vi "Get Reference for Demodulation.vi"(0 "AI Block Size":i32=5000, 1 "# channels":i32, 2 "Calculate REF?":bool, 5 "AI Rate":dbl=10000.0 format="%.2f", 7 "OSC Configuration":T3(array[cluster])=[[{"Signal Type"=enum."Sine Wave", "DC"=0.0, "Amplitude"=0.01, "frequency"=2.0, "Phase"=0.0}, {"Signal Type"=enum."Sine Wave", "DC"=0.0, "Amplitude"=0.01, "frequency"=2.0, "Phase"=0.0}], [{"Signal Type"=enum."Sine Wave", "DC"=0.0, "Amplitude"=0.01, "frequency"=2.0, "Phase"=0.0}, {"Signal Type"=enum."Sine Wave", "DC"=0.0, "Amplitude"=0.01, "frequency"=2.0, "Phase"=0.0}]] {"frequency" step=0.001 format="%.3p"; "Amplitude" format="%0.2p"; "DC" min=-0.99 max=0.99 format="%.2p"}, 9 "Phase&Tc":T1(array[cluster])=[{"Phase"=0.0, "Time constant"=0.1, "Set Tc"=FALSE, "Autophase"=FALSE, "Order"=2.0}, {"Phase"=0.0, "Time constant"=0.1, "Set Tc"=FALSE, "Autophase"=FALSE, "Order"=2.0}, {"Phase"=0.0, "Time constant"=0.1, "Set Tc"=FALSE, "Autophase"=FALSE, "Order"=2.0}, {"Phase"=0.0, "Time constant"=0.1, "Set Tc"=FALSE, "Autophase"=FALSE, "Order"=2.0}, {"Phase"=0.0, "Time constant"=0.1, "Set Tc"=FALSE, "Autophase"=FALSE, "Order"=2.0}, {"Phase"=0.0, "Time constant"=0.1, "Set Tc"=FALSE, "Autophase"=FALSE, "Order"=2.0}, {"Phase"=0.0, "Time constant"=0.1, "Set Tc"=FALSE, "Autophase"=FALSE, "Order"=2.0}, {"Phase"=0.0, "Time constant"=0.1, "Set Tc"=FALSE, "Autophase"=FALSE, "Order"=2.0}, {"Phase"=0.0, "Time constant"=0.1, "Set Tc"=FALSE, "Autophase"=FALSE, "Order"=2.0}, {"Phase"=0.0, "Time constant"=0.1, "Set Tc"=FALSE, "Autophase"=FALSE, "Order"=2.0}, {"Phase"=0.0, "Time constant"=0.1, "Set Tc"=FALSE, "Autophase"=FALSE, "Order"=2.0}, {"Phase"=0.0, "Time constant"=0.1, "Set Tc"=FALSE, "Autophase"=FALSE, "Order"=2.0}, {"Phase"=0.0, "Time constant"=0.1, "Set Tc"=FALSE, "Autophase"=FALSE, "Order"=2.0}] {"Phase" min=0.0 max=360.0 scale=0.0..360.0}, 11 "phase log":dbl[](array[numeric])=[0.99999999999938, 0.99999999999938], 12 "Results":dbl[][](array[numeric])=[[-0.007466313257110502, 0.006647442288790556, 0.009996715592438601, 138.3205414893834], [4.666416897873004e-05, 2.73365354254356e-05, 5.408170518337571e-05, 30.36238005772962], [4.0726992829495153e-05, 2.9330066584266565e-05, 5.01890501082782e-05, 35.760031216297186], [4.1405700938166546e-05, 2.8678109848811026e-05, 5.0367311370385436e-05, 34.706961203452664], [4.151375450731611e-05, 2.7252363446332437e-05, 4.965967304266818e-05, 33.28353283261694], [4.150189344545443e-05, 2.848421770375026e-05, 5.033644621695589e-05, 34.463187057405904]]) -> (6 "REF":T2(array[cluster]), 8 "Phase Log Out":dbl[](array[numeric]), 10 "Phase&Tc Out":T1(array[cluster]))   [LabVIEW 2013]
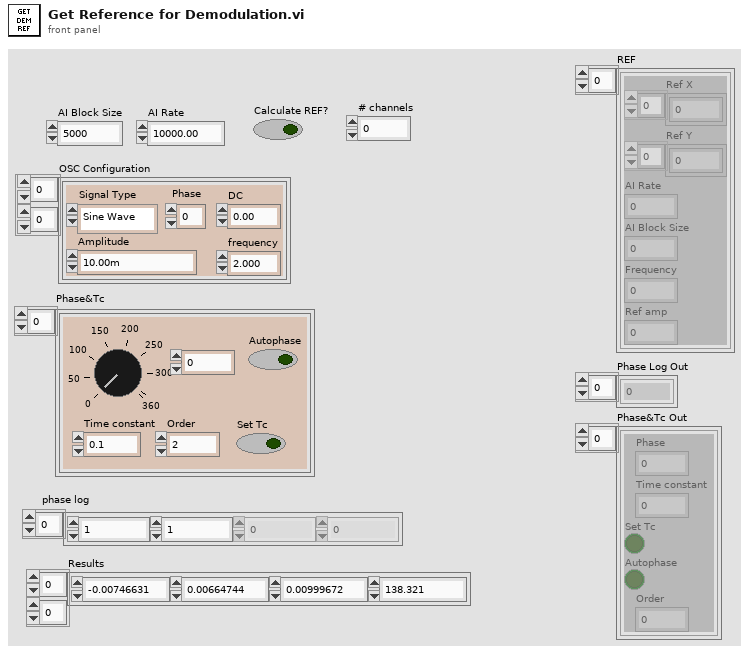
[diagram p1: front panel]
types:
  T1 = cluster{"Phase":dbl, "Time constant":dbl, "Set Tc":bool, "Autophase":bool, "Order":dbl}[]
  T2 = cluster{"Ref X":dbl[], "Ref Y":dbl[], "AI Rate":dbl, "AI Block Size":dbl, "Frequency":dbl, "Ref amp":dbl}[]
  T3 = cluster{"Signal Type":enum16{"Sine Wave", "Triangle Wave", "Square Wave", "Sawtooth Wave"}, "DC":dbl, "Amplitude":dbl, "frequency":dbl, "Phase":dbl}[][]
  T4 = cluster{"Signal Type":enum16{"Sine Wave", "Triangle Wave", "Square Wave", "Sawtooth Wave"}, "DC":dbl, "Amplitude":dbl, "frequency":dbl, "Phase":dbl}
  T5 = cluster{"Ref X":dbl[], "Ref Y":dbl[], "AI Rate":dbl, "AI Block Size":dbl, "Frequency":dbl, "Ref amp":dbl}
  T6 = cluster{"Phase":dbl, "Time constant":dbl, "Set Tc":bool, "Autophase":bool, "Order":dbl}
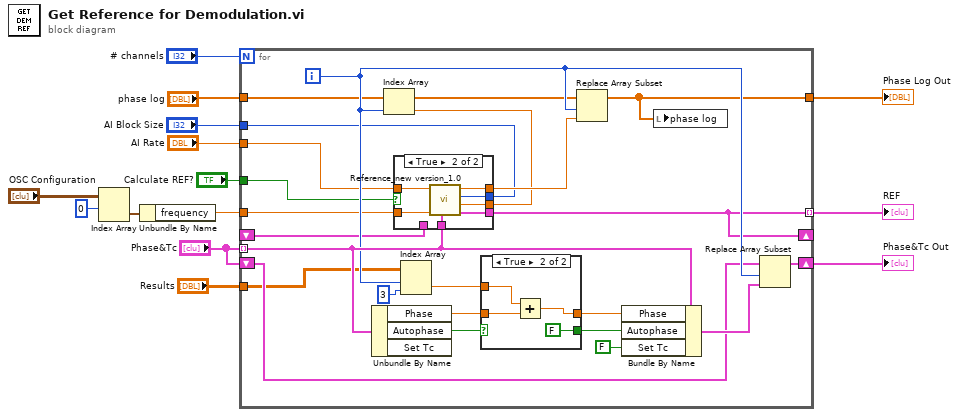
[diagram p0: block diagram]
diagram:
  w13 = 0 ("disabled index (col)")
  n1 = Index Array(array="OSC Configuration", index (row)=w13, index (col)=w13) -> (element=w6:T4)
  n2 = Unbundle By Name(w6) -> ("frequency"=w5:dbl)
  n3 = for {
    N: "# channels" -> [_]
    tunnel: "Phase&Tc" -> [w34] mode=indexing
    tunnel: [w20] -> w14 mode=indexing
    tunnel: "AI Block Size" -> [w26]
    tunnel: "AI Rate" -> [w25]
    tunnel: [w23] -> w9
    shift-right: [w22] -> w8
    shift-left: "Phase&Tc" -> [w21]
    shift-right: [w20] -> _
    shift-left: _ -> [w18]
    tunnel: w5 -> [w19]
    tunnel: "phase log" -> [w17]
    tunnel: "Results" -> [w16]
    tunnel: "Calculate REF?" -> [w15]
    i -> [w28]
    n4 = Unbundle By Name(w34) -> ("Phase"=w36:dbl, "Autophase"=w32:bool)  [unwired: 1 out]
    n5 = Index Array(array=w17, index=w28) -> (element=w24:dbl)
    n6 = case shown="True" w15 {
      tunnel: w34 -> [_ w46]
      tunnel: [w38 w45] -> w27
      tunnel: w26 -> [_ w44]
      tunnel: w25 -> [_ w43]
      tunnel: w24 -> [w38 w42]
      tunnel: [w39 w41] -> w20
      tunnel: w19 -> [_ w40]
      tunnel: w18 -> [w39 _]
      frame False {
      }
      frame True {
        n7 = call "Reference_new version_1.0.vi"("Phase log in"=w42, "AI Block Size"=w44, "Phase&time"=w46, "Frequency"=w40, "AI Rate"=w43) -> ("Ref out"=w41:T5, "Phase log"=w45:dbl)  [unwired: 3 in]
      }
    }
    n8 = Index Array(array=w16, index (row)=w28, index (col)=3 ("disabled index (col)")) -> (element=w35:dbl)
    n9 = case shown="True" w32 {
      selector: w32 -> [w47 _]
      tunnel: w36 -> [w48 w50]
      tunnel: w35 -> [_ w49]
      tunnel: [w48 w52] -> w33
      tunnel: [w47 FALSE] -> w31
      frame False {
      }
      frame True {
        n10 = Add(x=w49, y=w50) -> (x+y=w52:dbl)
      }
    }
    n11 = Replace Array Subset(array=w17, new element=w27, index=w28) -> (w23:dbl[])
    n12 = Bundle By Name(cluster=w34, "Phase"=w33, "Autophase"=w31, "Set Tc"=FALSE) -> (w30:T6)
    n13 = local write "phase log"(w23) -> ()
    n14 = Replace Array Subset(array=w21, new element=w30, index=w28) -> (w22:T1)
  }
  "REF" <- w14
  "Phase Log Out" <- w9
  "Phase&Tc Out" <- w8
